vi "Check Trigger Conditions.vi"(7 "Force Trigger?":bool caption="强制触发？", 8 "error in (no error)":errorcluster caption="错误输入（无错误）", 9 "Waveform Data":waveform(sgl)[](array[waveform]) caption="波形数据", 10 "Acquisition and Logging Configuration":T1={"Samples per Read"=100, "Number of Reads to Save"=20, "Number of Channels"=4, "Channel Scale Array"=[1.0, 1.0, 1.0, 1.0], "Channel Names"=[], "Trigger - RMS Value"=0.9999999999999994, "Trigger - Channel"=0, "Trigger - Time (Minute)"=10, "TDMS Properties"=[], "Data File Name"="cRIO_Data", "Date Rate"=20} caption="采集与记录配置" {"Date Rate" items=["51.200 kS/s (NI 9234)"=1, "25.600 kS/s (NI 9234)"=2, "17.067 kS/s (NI 9234)"=3, "12.80 kS/s (NI 9234)"=4, "10.240 kS/s (NI 9234)"=5, "8.533 kS/s (NI 9234)"=6, "7.314 kS/s (NI 9234)"=7, "6.400 kS/s (NI 9234)"=8, "5.689 kS/s (NI 9234)"=9, "5.120 kS/s (NI 9234)"=10, "4.654 kS/s (NI 9234)"=11, "4.267 kS/s (NI 9234)"=12, "3.938 kS/s (NI 9234)"=13, "3.657 kS/s (NI 9234)"=14, "3.413 kS/s (NI 9234)"=15, "3.200 kS/s (NI 9234)"=16, "3.012 kS/s (NI 9234)"=17, "2.845 kS/s (NI 9234)"=18, "2.695 kS/s (NI 9234)"=19, "2.560 kS/s (NI 9234)"=20, "2.438 kS/s (NI 9234)"=21, "2.328 kS/s (NI 9234)"=22, "2.226 kS/s (NI 9234)"=23, "2.133 kS/s (NI 9234)"=24, "2.048 kS/s (NI 9234)"=25, "1.969 kS/s (NI 9234)"=26, "1.896 kS/s (NI 9234)"=27, "1.829 kS/s (NI 9234)"=28, "1.765 kS/s (NI 9234)"=29, "1.707 kS/s (NI 9234)"=30, "1.652 kS/s (NI 9234)"=31]}) -> (0 "error out":errorcluster caption="错误输出", 3 "Trigger Condition Met?":bool caption="触发条件满足？")   [LabVIEW 2013]
uses:
  controls/Acquisition and Logging Configuration.ctl
  controls/TDMS Properties.ctl
  <vilib>/LabVIEW Targets/FPGA/cRIO/shared/nicrio_ModuleControls/nicrio_cRIO-9234_DataRatesRing2.ctl
  <vilib>/Analysis/5stat.llb/RMS (DBL).vi
  <vilib>/Analysis/NI_AALPro.lvlib
panel:
  # "通道"
  # "保存"
  # "采样"
  # "触发"
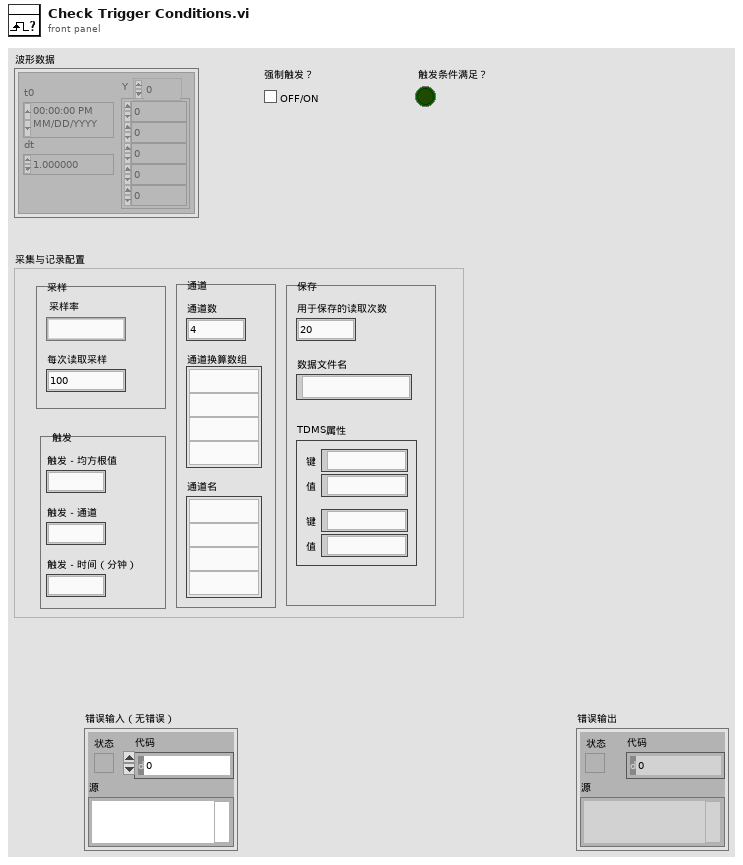
[diagram p1: front panel]
types:
  T1 = typedef "Acquisition and Logging Configuration.ctl" = cluster{"Samples per Read":i32, "Number of Reads to Save":i32, "Number of Channels":i32, "Channel Scale Array":fxp<+,24,12>[], "Channel Names":string[], "Trigger - RMS Value":dbl, "Trigger - Channel":i32, "Trigger - Time (Minute)":i32, "TDMS Properties":T2[], "Data File Name":string, "Date Rate":T3}
  T2 = typedef "TDMS Properties.ctl" = cluster{"Name":string, "Value":string}
  T3 = typedef "nicrio_cRIO-9234_DataRatesRing2.ctl" = u16
  T4 = typedef "LVDateTimeRec.ctl" = cluster{"fractional second":dbl, "second":i32, "minute":i32, "hour":i32, "day of month":i32, "month":i32, "year":i32, "day of week":i32, "day of year":i32, "DST":i32}
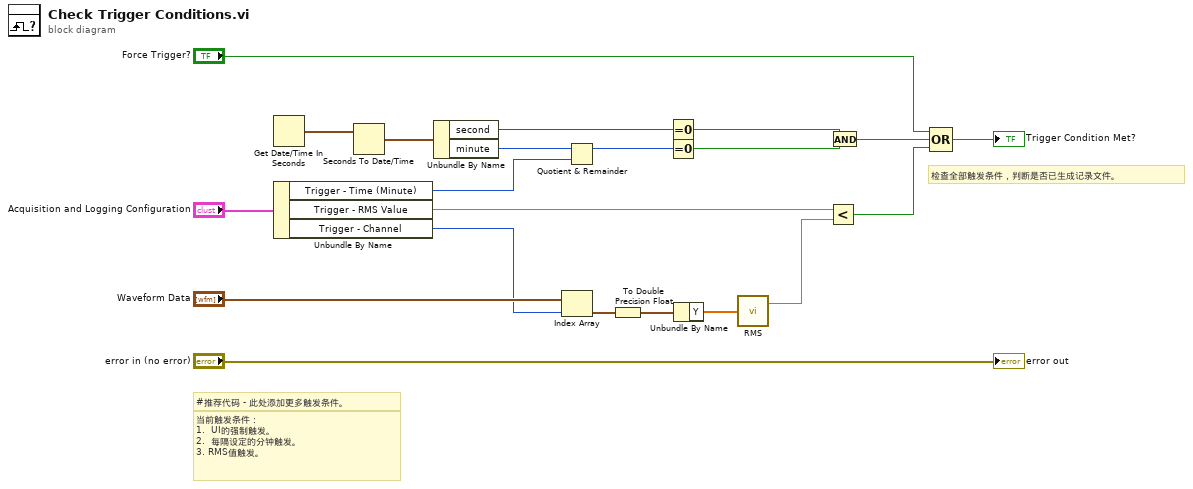
[diagram p0: block diagram]
diagram:
  # "检查全部触发条件，判断是否已生成记录文件。"
  # "当前触发条件：\n1.  UI的强制触发。\n2.  每隔设定的分钟触发。\n3. RMS值触发。"
  # "#推荐代码 - 此处添加更多触发条件。"
  n1 = Get Date/Time In Seconds() -> (seconds since 1Jan1904=w7:timestamp)
  n2 = Unbundle By Name("Acquisition and Logging Configuration") -> ("Trigger - Time (Minute)"=w5:i32, "Trigger - RMS Value"=w18:dbl, "Trigger - Channel"=w17:i32)
  n3 = Seconds To Date/Time(time stamp (now)=w7) -> (date time rec=w13:T4)  [unwired: 1 out]
  n4 = Unbundle By Name(w13) -> ("second"=w12:i32, "minute"=w11:i32)
  n5 = Index Array(array="Waveform Data", index=w17) -> (element=w16:waveform(sgl))
  n6 = Quotient & Remainder(x=w11, y=w5) -> (x-y*floor(x/y)=w10:i32)  [unwired: 1 out]
  n7 = To Double Precision Float(number=w16) -> (double precision float=w15:waveform(dbl))
  n8 = Equal To 0?(x=w12) -> (x = 0?=w9:bool)
  n9 = Equal To 0?(x=w10) -> (x = 0?=w8:bool)
  n10 = Unbundle By Name(w15) -> ("Y"=w3:dbl[])
  n11 = call-poly <vilib>:"RMS.vi"("X"=w3) -> ("rms value"=w2:dbl)  [unwired: 1 out]
  n12 = Less?(x=w18, y=w2) -> (x < y?=w14:bool)
  n13 = And(x=w9, y=w8) -> (x .and. y?=w4:bool)
  n14 = Compound Arithmetic op=OR("Force Trigger?", w4, w14) -> (→"Trigger Condition Met?":bool)
  "error out" <- "error in (no error)"
